vi "RemoteControl.vi"() -> ()   [LabVIEW 2019]
uses:
  <vilib>/ReMiSYS/ReMiSYS_WSCbot-XS/SubVI/XS_F710.ctl
  <vilib>/ReMiSYS/ReMiSYS_WSCbot-XS/SubVI/XS_stick.ctl
  <vilib>/ReMiSYS/ReMiSYS_WSCbot-XS/SubVI/XS_gamepadF710.lvclass
  WSCbot_V3_Toolkit.lvlibp/WSCBOTV3_Toolkit/IO/LowLevel/PulseCounter.ctl
  <vilib>/Platform/TimedLoop/XDataNode/timing_clust.ctl
  <vilib>/Platform/TimedLoop/XDataNode/nitl_modes.ctl
  <vilib>/Platform/TimedLoop/XDataNode/wakeup.ctl
  WSCbot_V3_Toolkit.lvlibp/WSCBOTV3_Toolkit/IO/LowLevel/IO_Chanel_DIO.ctl
  <vilib>/platform/TimedLoop/XDataNode/XDataNode.xnode
  <vilib>/Platform/TimedLoop/XDataNode/XDNodeRunTimeDep.lvlib
  WSCbot_V3_Toolkit.lvlibp
panel:
  out "PulseCount":i32
  out "Trun 180":bool
  out "positive":bool
  out "F710 button info.right":bool
  out "F710 button info.left":bool
  out "Angle_index":i32
  in  "Angle_array(deg)":dbl[](array[numeric])=[-65.0, 25.0, 115.0]
  out "F710 button info.LogiB":bool
  out "F710 button info.rightStick":bool
  out "EMS":bool
  in  "MaxSpeed":dbl=800.0
  out "H/L Speed":bool
  out "Current_High":dbl
  out "F710 button info.down":bool
  out "F710 button info.up":bool
  out "Flat":bool
  out "Home?":bool
  out "leftStick_Touch\nTimes":i8
  in  "High_array(mm)":dbl[](array[numeric])=[0.0, 78.0, 128.0, 250.0, 300.0]
  out "Hight":i32
  out "Front/Back":bool
  out "up":bool
  out "F710 button info.leftStick":bool
  out "F710 button info.B":bool
  out "F710 button info.X":bool
  out "F710 button info.A":bool
  out "F710 button info.Y":bool
  out "F710 button info.RB":bool
  out "F710 button info.LB":bool
  out "ini":bool
  out "reset":bool
  out "angle":dbl
  out "speed":dbl
  out "Error Out":errorcluster
  in  "Stop Button":bool
  in  "error in (no error)":errorcluster
  in  "INPUT S/N":string="U16N121E"
  in  "VISA resource name":refnum<visa-resource-name>="USB0::0x046D::0xC21F::145C9E1C::RAW"
  out "Stop Output":bool
  out "SpeedArray":dbl[](array[numeric])
  out "F710":T1
  # "螺絲物料櫃(1)\n螺絲物料櫃(2)\n螺帽物料櫃\n螺帽物料櫃瞄準"
  # "總高度300mm"
  # "朝左"
  # "朝前"
  # "朝右"
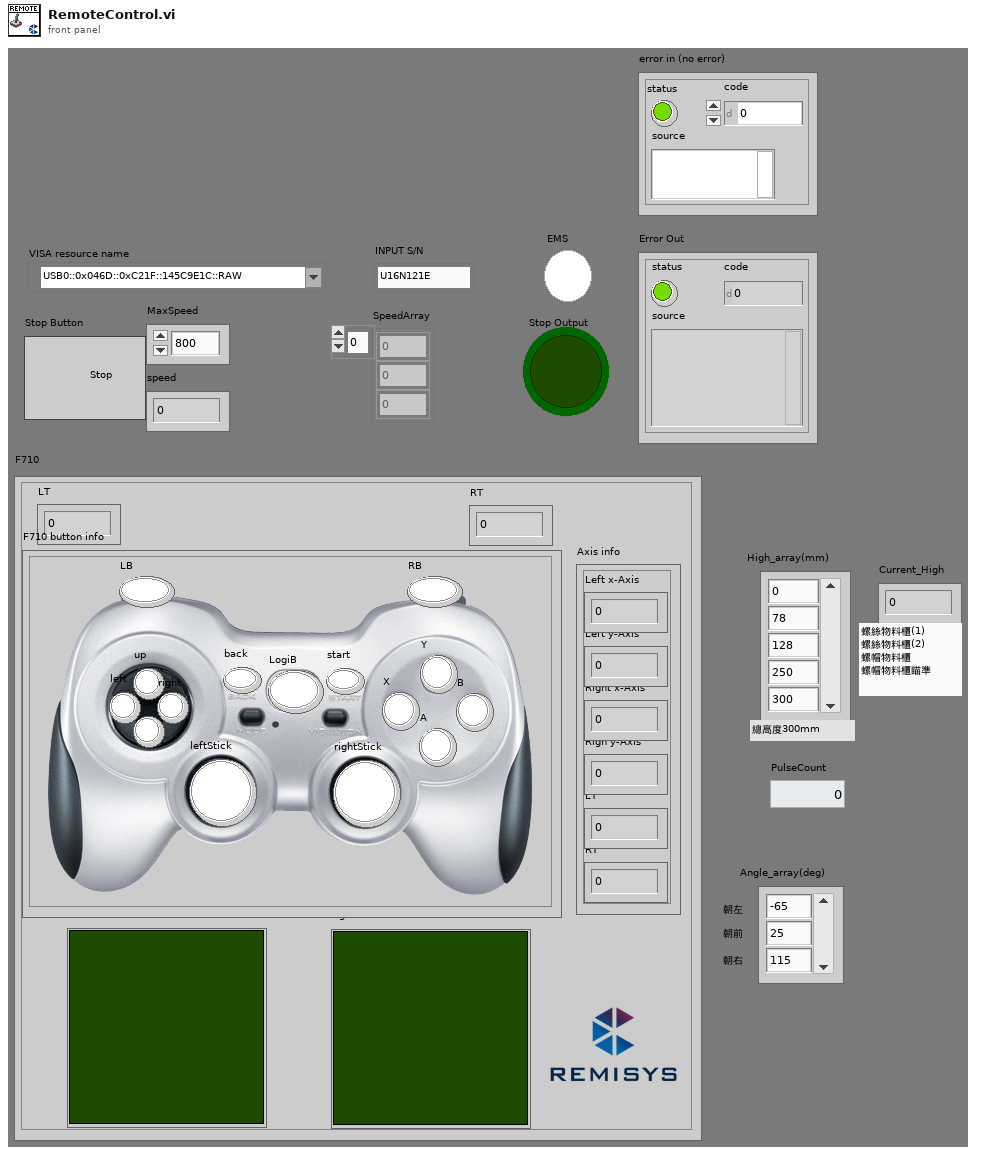
[diagram p1: front panel]
types:
  T1 = typedef "XS_F710.ctl" = cluster{"RT":u8, "LT":u8, "RightStick":T2, "LeftStick":T2, "Axis info":cluster{"Left x-Axis":i8, "Left y-Axis":i8, "Right x-Axis":i8, "Righ y-Axis":i8, "LT":u8, "RT":u8}, "F710 button info":cluster{"RB":bool, "LB":bool, "rightStick":bool, "leftStick":bool, "start":bool, "back":bool, "right":bool, "left":bool, "down":bool, "up":bool, "Y":bool, "X":bool, "B":bool, "A":bool, "LogiB":bool}}
  T2 = typedef "XS_stick.ctl" = cluster{"X":dbl, "Y":dbl}[]
  T3 = typedef "WSCbot_V3_Toolkit.lvlibp/PulseCounter.ctl" = enum16{"CH1", "CH2", "CH3", "CH4", "CH5"}
  T4 = typedef "WSCbot_V3_Toolkit.lvlibp/IO_Chanel_DIO.ctl" = enum16{"A/DIO9", "A/DIO10", "C/DIO0", "C/DIO1", "C/DIO2", "C/DIO3", "C/DIO4", "C/DIO5", "C/DIO6"}
  T5 = typedef "XDNodeRunTimeDep.lvlib/timing_clust.ctl" = cluster{"Expected End [f-1]":u64, "Actual End [f-1]":u64, "Finished Late? [f-1]":bool, "Expected End [i-1]":u64, "Actual End [i-1]":u64, "Finished Late? [i-1]":bool, "Expected Start [i]":u64, "Actual Start [i]":u64, "Expected Start [f]":u64, "Actual Start [f]":u64, "Source Name":string, "Structure Name":string, "Period":i64, "Deadline":i64, "Offset":i64, "Start":i64, "Priority":i32, "Timeout":i32, "Mode":T6, "Wakeup Reason":T7, "Error":errorcluster, "Source Type":string, "Secondary Source Type":string, "Global End Time":u64, "Global Start Time":u64, "Frame Duration":u64, "Iteration Duration":u64, "Assigned CPU":i32, "I/O Scan Engine Mode":u32}
  T6 = typedef "XDNodeRunTimeDep.lvlib/nitl_modes.ctl" = enum32{"No Change", "Process missed periods, maintain original phase", "Discard missed periods, maintain original phase", "Process missed periods, ignore original phase", "Discard missed periods, ignore original phase"}
  T7 = typedef "XDNodeRunTimeDep.lvlib/wakeup.ctl" = enum32{"Normal", "Aborted", "Asynchronous wakeup", "Timing source error", "Timed loop error", "Timeout"}
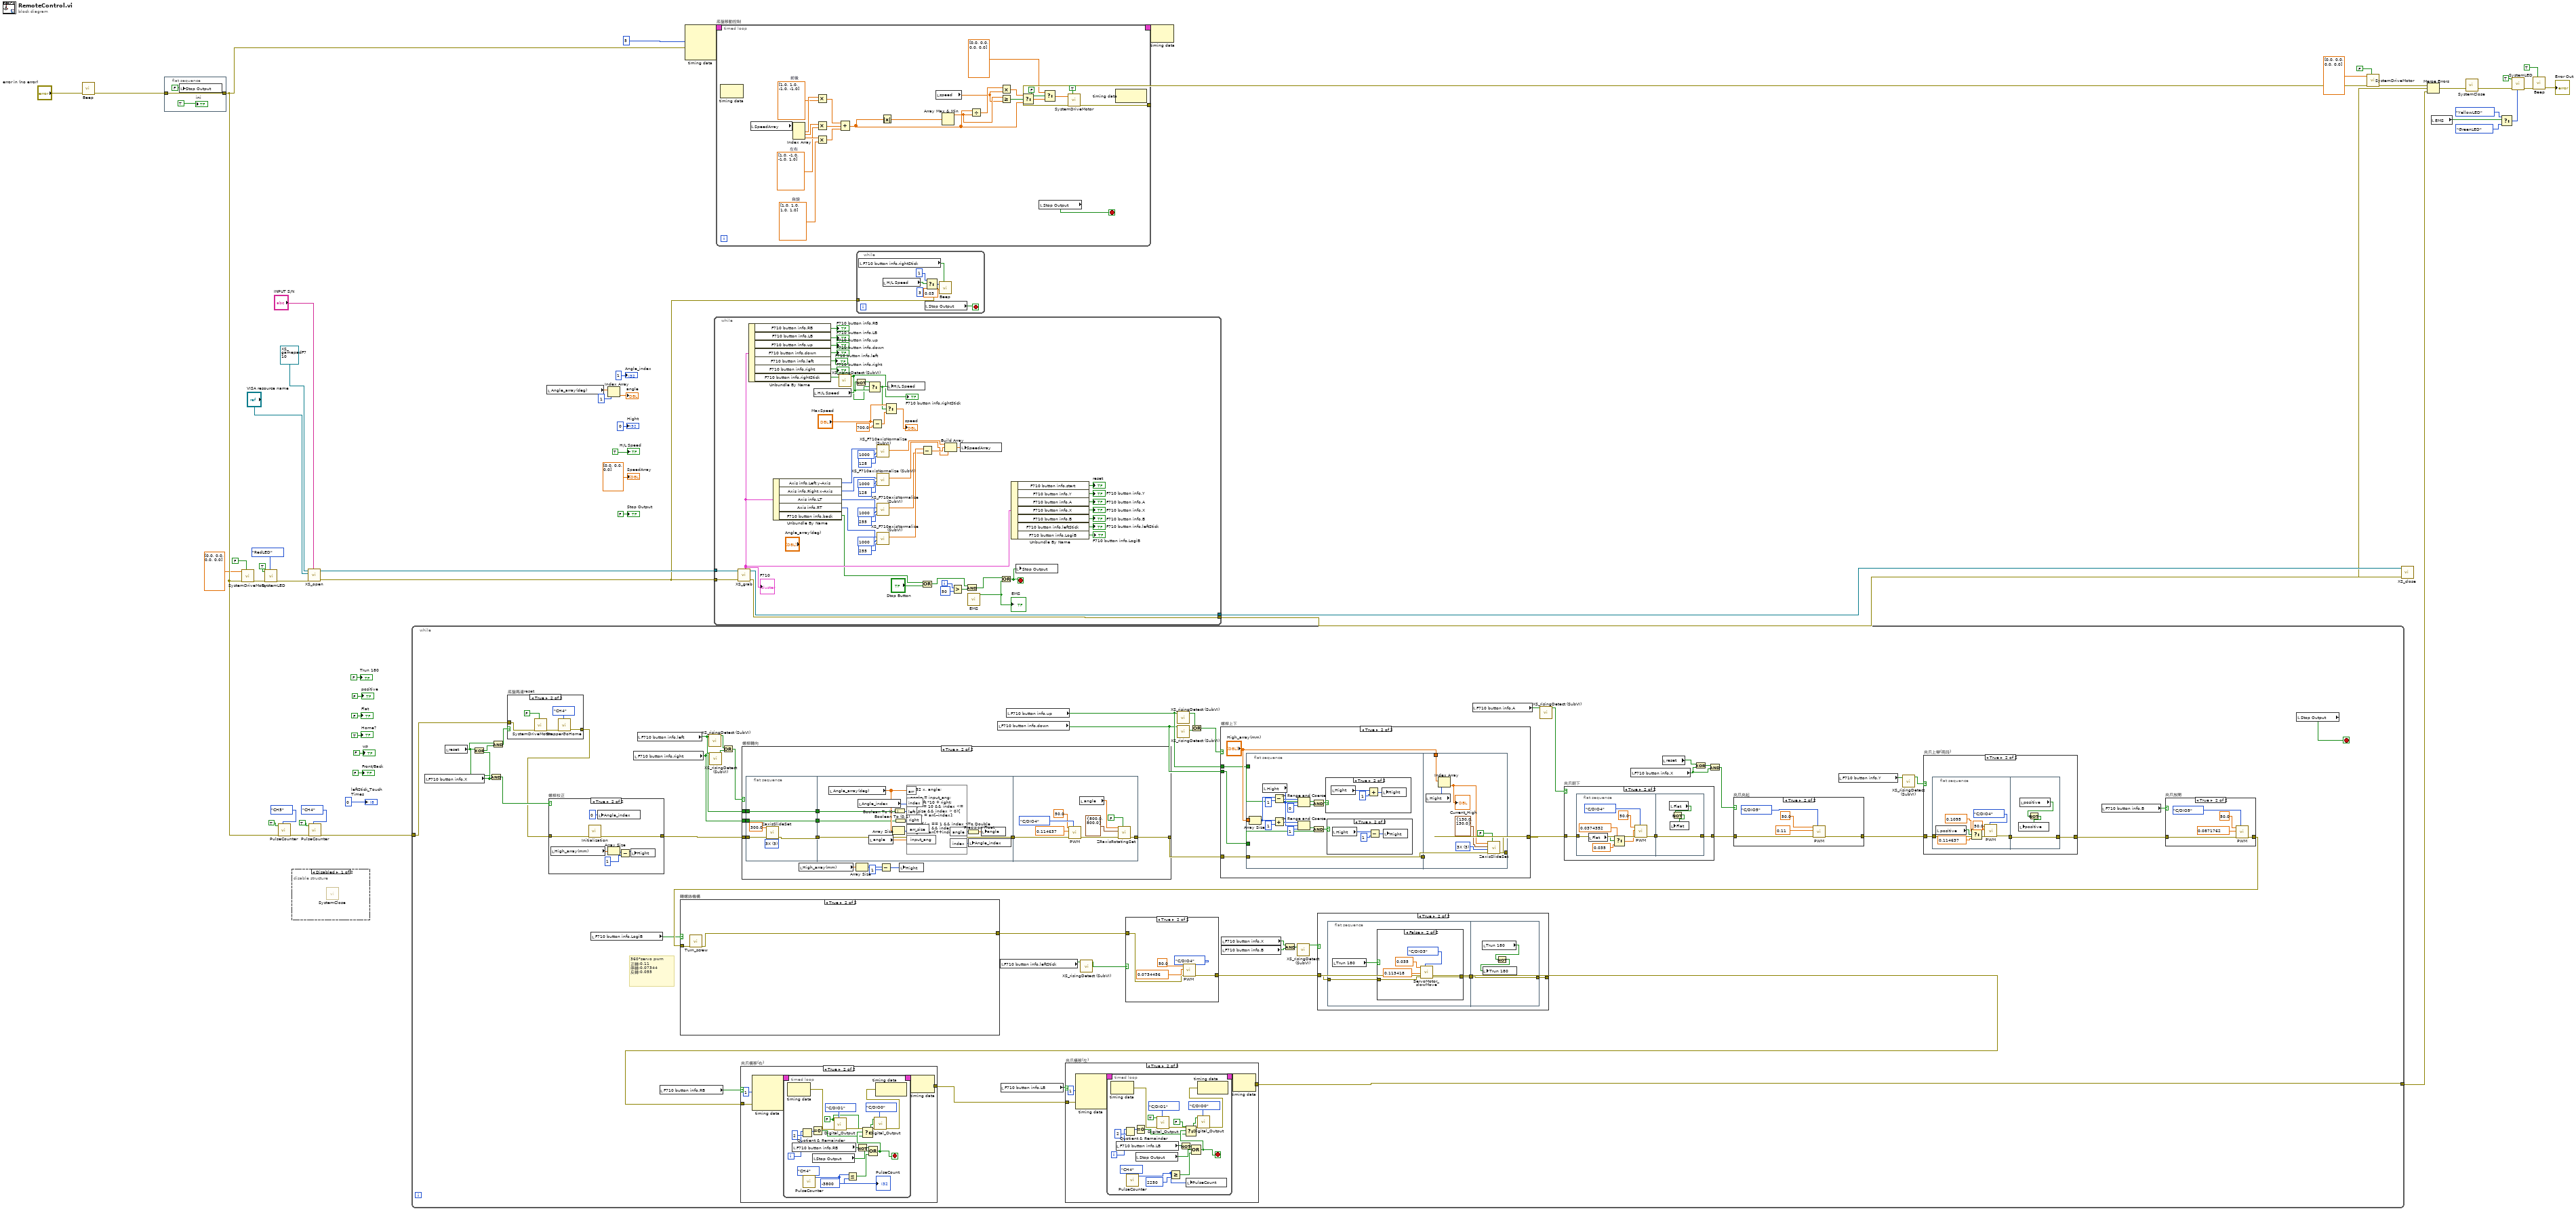
[diagram p0: block diagram]
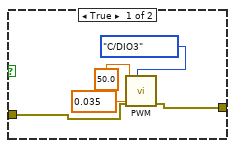
[diagram p4: hidden frame]
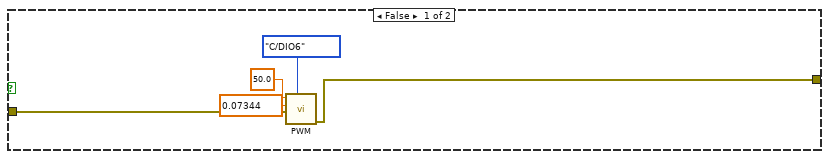
[diagram p8: hidden frame]
diagram:
  n1 = call "Beep.vi"("Error In"="error in (no error)") -> ("Error Out"=w17:errorcluster)  [unwired: 10 in]
  n2 = flat-sequence {
    tunnel: [w58] -> w35
    tunnel: w17 -> [w58]
    frame #0 {
      n3 = local write "Stop Output"(FALSE ("Stop Output")) -> ()
      "ini" <- TRUE
    }
  }
  n4 = call "SystemDriveMotor.vi"("Enable?"=FALSE, "error in"=w35, "4xMotor(deg/s)"=dbl[] [0.0, 0.0, 0.0, 0.0]) -> ("error out"=w46:errorcluster)  [unwired: 7 in, 1 out]
  n5 = call "SystemLED.vi"("SelectColor"=enum16{"RedLED", "GreenLED", "YellowLED"}."RedLED", "error in"=w46, "Set"=TRUE) -> ("error out"=w49:errorcluster)  [unwired: 8 in]
  n6 = call "PulseCounter.vi"("PulseCounterChanel"=PulseCounter."CH5", "error in"=w35, "Reset"=TRUE) -> ("error out"=w31:errorcluster)  [unwired: 7 in, 1 out]
  n7 = disable-structure shown="Disabled" {
    frame Disabled {
      n8 = call "SystemClose.vi"() -> ()  [unwired: 3 in, 1 out]
    }
    frame Enabled {
    }
  }
  n9 = call <vilib>:"XS_open.vi"("INPUT S/N"="INPUT S/N", "error in (no error)"=w49, "VISA resource name"="VISA resource name", "gamepadF710 in"=refnum<class "XS_gamepadF710.lvclass"> refnum) -> ("error out"=w14:errorcluster, "gamepadF710 out"=w50:refnum<class "XS_gamepadF710.lvclass">)  [unwired: 6 in]
  n10 = call "PulseCounter.vi"("PulseCounterChanel"=PulseCounter."CH4", "error in"=w31, "Reset"=TRUE) -> ("error out"=w30:errorcluster)  [unwired: 7 in, 1 out]
  n11 = while {
    tunnel: w30 -> [w94]
    tunnel: [w60] -> w36
    stop <- w106 stop-if-true
    # "360°servo pwm\n正轉:0.11\n停轉:0.07344\n反轉:0.055"
    n12 = local read "F710 button info.X"() -> (w103:bool)
    n13 = local read "reset"() -> (w86:bool)
    n14 = Exclusive Or(1:w103, 2:w86) -> (0:w87:bool)
    n15 = And(x=w86, y=w103) -> (x .and. y?=w104:bool)
    n16 = And(x=w86, y=w87) -> (x .and. y?=w88:bool)
    n17 = case "底盤馬達reset" shown="True" w88 {
      tunnel: w94 -> [w255 w257]
      tunnel: [w255 w256] -> w93
      frame False {
      }
      frame True {
        n18 = call "SystemDriveMotor.vi"("Enable?"=FALSE, "error in"=w257) -> ("error out"=w259:errorcluster)  [unwired: 8 in, 1 out]
        n19 = call "StepperGoHome.vi"("PulseCounterChanel"=PulseCounter."CH4", "Error In"=w259) -> ("Error Out"=w256:errorcluster)  [unwired: 7 in, 2 out]
      }
    }
    n20 = case "螺桿校正" shown="True" w104 {
      tunnel: w93 -> [w261 w268]
      tunnel: [w261 w266] -> w105
      frame False {
      }
      frame True {
        n21 = local read "High_array(mm)"() -> (w265:dbl[])
        n22 = call "Initialization.vi"("Error In"=w268) -> ("Error Out"=w266:errorcluster)  [unwired: 10 in]
        n23 = local write "Angle_index"(0 ("Hight")) -> ()
        n24 = Array Size(array=w265) -> (size(s)=w264:i32)
        n25 = Subtract(x=w264, y=1) -> (x-y=w262:i32)
        n26 = local write "Hight"(w262) -> ()
      }
    }
    n27 = local read "F710 button info.LogiB"() -> (w75:bool)
    n28 = local read "F710 button info.right"() -> (w70:bool)
    n29 = local read "F710 button info.left"() -> (w69:bool)
    n30 = local read "F710 button info.RB"() -> (w78:bool)
    n31 = call <vilib>:"XS_risingDetect (SubVI).vi"("y"=w69) -> ("Boolean"=w73:bool)  [unwired: 10 in]
    n32 = call <vilib>:"XS_risingDetect (SubVI).vi"("y"=w70) -> ("Boolean"=w72:bool)  [unwired: 10 in]
    n33 = Or(x=w73, y=w72) -> (x .or. y?=w71:bool)
    n34 = case "螺桿轉向" shown="True" w71 {
      tunnel: w105 -> [w306 w318]
      tunnel: [w306 w313] -> w99
      tunnel: w70 -> [_ w310]
      tunnel: w69 -> [_ w307]
      frame False {
      }
      frame True {
        n35 = flat-sequence {
          tunnel: w318 -> [w322]
          tunnel: [w319] -> w312
          tunnel: w310 -> [w321]
          tunnel: [w321] -> w309
          tunnel: [w320] -> w308
          tunnel: w307 -> [w320]
          tunnel: w312 -> [w336]
          tunnel: [w336] -> w311
          tunnel: w309 -> [w326]
          tunnel: w308 -> [w325]
          tunnel: w311 -> [w342]
          tunnel: [w338] -> w313
          frame #0 {
            w323 = u16 3 items=["0X", "1X", "2X", "3X"] ("findHomeVel (times)")
            n36 = call "ZaxisSlideSet.vi"("error in"=w322, "findHomeVel (times)"=w323, "TargetABSHight(mm)"=300.0) -> ("error out"=w319:errorcluster)  [unwired: 7 in, 1 out]
          }
          frame #1 {
            n37 = local read "Angle_array(deg)"() -> (w332:dbl[])
            n38 = local read "Angle_index"() -> (w333:i32)
            n39 = local read "angle"() -> (w327:dbl)
            n40 = Array Size(array=w332) -> (size(s)=w329:i32)
            n41 = Boolean To (0,1)(Boolean=w325) -> (0, 1=w335:i16)
            n42 = Boolean To (0,1)(Boolean=w326) -> (0, 1=w334:i16)
            n43 = formula code="int32 x, angle;\n\nangle = input_ang;\nx = left *10 + right;\nif (x == 10 && index <= arr_size && index > 0){\nangle = arr[--index];\n}\nelse if ( x == 1 && index < arr_size-1 && index >=0){\nangle = arr[++index];\n}"("left"=w335, "right"=w334, "index"=w333, "arr"=w332, "arr_size"=w329, "input_ang"=w327) -> ("angle"=w330:i32, "index"=w328:i32)
            n44 = To Double Precision Float(number=w330) -> (double precision float=w331:dbl)
            n45 = local write "Angle_index"(w328) -> ()
            n46 = local write "angle"(w331) -> ()
          }
          frame #2 {
            n47 = call "PWM.vi"("IO_Chanel"=IO_Chanel_DIO."C/DIO4", "error in"=w342, "DutyCycle"=0.114637, "Frequency(Hz)"=50.0) -> ("error out"=w341:errorcluster)  [unwired: 7 in]
            n48 = local read "angle"() -> (w337:dbl)
            n49 = call "ZRaxisRotatingSet.vi"("Reset"=FALSE, "error in"=w341, "Velocity(deg/s)&ACC(deg/ss)"=cluster{"Velocity(cm/s)":dbl, "ACC(cm/ss)":dbl} {"Velocity(cm/s)"=800.0, "ACC(cm/ss)"=800.0}, "TargetHight(deg)"=w337) -> ("error out"=w338:errorcluster)  [unwired: 6 in, 1 out]
          }
        }
        n50 = local read "High_array(mm)"() -> (w317:dbl[])
        n51 = Array Size(array=w317) -> (size(s)=w316:i32)
        n52 = Subtract(x=w316, y=1) -> (x-y=w314:i32)
        n53 = local write "Hight"(w314) -> ()
      }
    }
    n54 = local read "F710 button info.down"() -> (w79:bool)
    n55 = local read "F710 button info.leftStick"() -> (w68:bool)
    n56 = local read "F710 button info.LB"() -> (w77:bool)
    n57 = local read "F710 button info.up"() -> (w80:bool)
    n58 = call <vilib>:"XS_risingDetect (SubVI).vi"("y"=w68) -> ("Boolean"=w67:bool)  [unwired: 10 in]
    n59 = call <vilib>:"XS_risingDetect (SubVI).vi"("y"=w80) -> ("Boolean"=w76:bool)  [unwired: 10 in]
    n60 = call <vilib>:"XS_risingDetect (SubVI).vi"("y"=w79) -> ("Boolean"=w81:bool)  [unwired: 10 in]
    n61 = Or(x=w76, y=w81) -> (x .or. y?=w74:bool)
    n62 = case "螺桿上下" shown="True" w74 {
      tunnel: [w269 w273] -> w98
      tunnel: w99 -> [w269 w275]
      tunnel: w80 -> [_ w271]
      tunnel: w79 -> [_ w270]
      frame False {
      }
      frame True {
        n63 = flat-sequence {
          tunnel: "High_array(mm)" -> [w279]
          tunnel: w275 -> [w278]
          tunnel: [w278] -> w274
          tunnel: w271 -> [w277]
          tunnel: w270 -> [w276]
          tunnel: w274 -> [w300]
          tunnel: [w299] -> w273
          tunnel: "High_array(mm)" -> [w298]
          frame #0 {
            n64 = Array Size(array=w279) -> (size(s)=w289:i32)
            n65 = local read "Hight"() -> (w286:i32)
            n66 = Subtract(x=w289, y=1) -> (x-y=w291:i32)
            n67 = Add(x=w289, y=1) -> (x+y=w287:i32)
            n68 = In Range and Coerce(upper limit=w291, x=w286, lower limit=0) -> (In Range?=w285:bool)  [unwired: 1 out]
            n69 = In Range and Coerce(upper limit=w287, x=w286, lower limit=1) -> (In Range?=w283:bool)  [unwired: 1 out]
            n70 = And(x=w277, y=w285) -> (x .and. y?=w282:bool)
            n71 = And(x=w283, y=w276) -> (x .and. y?=w281:bool)
            n72 = case shown="True" w282 {
              frame False {
              }
              frame True {
                n73 = local read "Hight"() -> (w294:i32)
                n74 = Add(x=w294, y=1) -> (x+y=w293:i32)
                n75 = local write "Hight"(w293) -> ()
              }
            }
            n76 = case shown="True" w281 {
              frame False {
              }
              frame True {
                n77 = local read "Hight"() -> (w297:i32)
                n78 = Subtract(x=w297, y=1) -> (x-y=w296:i32)
                n79 = local write "Hight"(w296) -> ()
              }
            }
          }
          frame #1 {
            w302 = u16 3 items=["0X", "1X", "2X", "3X"] ("findHomeVel (times)")
            n80 = local read "Hight"() -> (w304:i32)
            n81 = Index Array(array=w298, index=w304) -> (element=w305:dbl)
            "Current_High" <- w305
            n82 = call "ZaxisSlideSet.vi"("Reset"=FALSE, "error in"=w300, "findHomeVel (times)"=w302, "Velocity(mm/s)&ACC(mm/ss)"=cluster{"Velocity(cm/s)":dbl, "ACC(cm/ss)":dbl} {"Velocity(cm/s)"=130.0, "ACC(cm/ss)"=130.0}, "TargetABSHight(mm)"=w305) -> ("error out"=w299:errorcluster)  [unwired: 5 in, 1 out]
          }
        }
      }
    }
    n83 = local read "F710 button info.X"() -> (w64:bool)
    n84 = local read "F710 button info.B"() -> (w63:bool)
    n85 = And(x=w64, y=w63) -> (x .and. y?=w62:bool)
    n86 = call <vilib>:"XS_risingDetect (SubVI).vi"("y"=w62) -> ("Boolean"=w61:bool)  [unwired: 10 in]
    n87 = local read "F710 button info.A"() -> (w83:bool)
    n88 = call <vilib>:"XS_risingDetect (SubVI).vi"("y"=w83) -> ("Boolean"=w82:bool)  [unwired: 10 in]
    n89 = case "夾爪朝下" shown="True" w82 {
      tunnel: [w225 w228] -> w101
      tunnel: w98 -> [w225 w227]
      frame False {
      }
      frame True {
        n90 = flat-sequence {
          tunnel: w227 -> [w233]
          tunnel: [w234] -> w226
          tunnel: [w239] -> w228
          tunnel: w226 -> [w239]
          frame #0 {
            n91 = local read "Flat"() -> (w230:bool)
            n92 = Select(t=0.0374352, s=w230, f=0.035 ("DutyCycle")) -> (s? t:f=w231:dbl)
            n93 = call "PWM.vi"("IO_Chanel"=IO_Chanel_DIO."C/DIO4", "error in"=w233, "DutyCycle"=w231, "Frequency(Hz)"=50.0) -> ("error out"=w234:errorcluster)  [unwired: 7 in]
          }
          frame #1 {
            n94 = local read "Flat"() -> (w237:bool)
            n95 = Not(x=w237) -> (.not. x?=w238:bool)
            n96 = local write "Flat"(w238) -> ()
          }
        }
      }
    }
    n97 = local read "F710 button info.X"() -> (w90:bool)
    n98 = local read "reset"() -> (w89:bool)
    n99 = Exclusive Or(1:w90, 2:w89) -> (0:w92:bool)
    n100 = And(x=w92, y=w90) -> (x .and. y?=w91:bool)
    n101 = case "夾爪夾起" shown="True" w91 {
      tunnel: w101 -> [w213 w215]
      tunnel: [w213 w214] -> w97
      frame False {
      }
      frame True {
        n102 = call "PWM.vi"("IO_Chanel"=IO_Chanel_DIO."C/DIO5", "error in"=w215, "DutyCycle"=0.11, "Frequency(Hz)"=50.0) -> ("error out"=w214:errorcluster)  [unwired: 7 in]
      }
    }
    n103 = local read "F710 button info.Y"() -> (w85:bool)
    n104 = call <vilib>:"XS_risingDetect (SubVI).vi"("y"=w85) -> ("Boolean"=w84:bool)  [unwired: 10 in]
    n105 = case "夾爪上舉(兩段)" shown="True" w84 {
      tunnel: [w240 w242] -> w102
      tunnel: w97 -> [w240 w243]
      frame False {
      }
      frame True {
        n106 = flat-sequence {
          tunnel: w243 -> [w249]
          tunnel: [w248] -> w241
          tunnel: [w254] -> w242
          tunnel: w241 -> [w254]
          frame #0 {
            n107 = local read "positive"() -> (w245:bool)
            n108 = Select(t=0.1095 ("DutyCycle"), s=w245, f=0.114637 ("DutyCycle")) -> (s? t:f=w247:dbl)
            n109 = call "PWM.vi"("IO_Chanel"=IO_Chanel_DIO."C/DIO4", "error in"=w249, "DutyCycle"=w247, "Frequency(Hz)"=50.0) -> ("error out"=w248:errorcluster)  [unwired: 7 in]
          }
          frame #1 {
            n110 = local read "positive"() -> (w253:bool)
            n111 = Not(x=w253) -> (.not. x?=w252:bool)
            n112 = local write "positive"(w252) -> ()
          }
        }
      }
    }
    n113 = local read "F710 button info.B"() -> (w100:bool)
    n114 = case "夾爪放開" shown="True" w100 {
      tunnel: w102 -> [w219 w221]
      tunnel: [w219 w220] -> w96
      frame False {
      }
      frame True {
        n115 = call "PWM.vi"("IO_Chanel"=IO_Chanel_DIO."C/DIO5", "error in"=w221, "DutyCycle"=0.0871762, "Frequency(Hz)"=50.0) -> ("error out"=w220:errorcluster)  [unwired: 7 in]
      }
    }
    n116 = case "轉螺絲機構" shown="True" w75 {
      tunnel: w96 -> [w207 w212]
      tunnel: [w206 w211] -> w66
      frame False {
        n117 = call "PWM.vi"("IO_Chanel"=IO_Chanel_DIO."C/DIO6", "error in"=w207, "DutyCycle"=0.07344, "Frequency(Hz)"=50.0) -> ("error out"=w206:errorcluster)  [unwired: 7 in]
      }
      frame True {
        n118 = call "Turn_screw.vi"("Error In"=w212) -> ("Error Out"=w211:errorcluster)  [unwired: 10 in]
      }
    }
    n119 = case shown="True" w67 {
      tunnel: w66 -> [w127 w130]
      tunnel: [w127 w129] -> w65
      frame False {
      }
      frame True {
        n120 = call "PWM.vi"("IO_Chanel"=IO_Chanel_DIO."C/DIO4", "error in"=w130, "DutyCycle"=0.0734456, "Frequency(Hz)"=50.0) -> ("error out"=w129:errorcluster)  [unwired: 7 in]
      }
    }
    n121 = case "夾爪橫移(右)" shown="True" w78 {
      tunnel: w65 -> [w170 w172]
      tunnel: [w170 w171] -> w95
      frame False {
      }
      frame True {
        n122 = node-c288(i64 1 ("Period"), w172) -> (w175:T5)  [unwired: 2 in]
        n123 = timed-loop {
          timing: w175 -> [_]
          timing-out: [_] -> w174
          i -> [w189]
          stop <- w179 stop-if-true
          w177 = FALSE ("False/True")
          n124 = node-c288() -> (w185:errorcluster)  [unwired: 1 in]
          n125 = local read "F710 button info.RB"() -> (w188:bool)
          n126 = Quotient & Remainder(x=w189, y=2) -> (x-y*floor(x/y)=w190:i32)  [unwired: 1 out]
          n127 = call "PulseCounter.vi"("PulseCounterChanel"=PulseCounter."CH4") -> ("PulseCount"=w182:i32)  [unwired: 9 in, 1 out]
          "PulseCount" <- w182
          n128 = Equal To 0?(x=w190) -> (x = 0?=w178:bool)
          n129 = local read "Stop Output"() -> (w186:bool)
          n130 = call "Digital_Output.vi"("IO_Chanel"=IO_Chanel_DIO."C/DIO1", "error in"=w185, "False/True"=w177) -> ("error out"=w193:errorcluster)  [unwired: 8 in]
          n131 = Less Or Equal?(x=w182, y=-3800) -> (x <= y?=w180:bool)
          n132 = Not(x=w188) -> (.not. x?=w187:bool)
          n133 = Compound Arithmetic op=OR(w187, w186, w180) -> (w179:bool)
          n134 = Select(t=w177, s=w179, f=w178) -> (s? t:f=w176:bool)
          n135 = call "Digital_Output.vi"("IO_Chanel"=IO_Chanel_DIO."C/DIO0", "error in"=w193, "False/True"=w176) -> ("error out"=w184:errorcluster)  [unwired: 8 in]
          n136 = node-c288(w184) -> ()  [unwired: 1 out]
        }
        n137 = node-c288(w174) -> (w171:errorcluster)
      }
    }
    n138 = case "夾爪橫移(左)" shown="True" w77 {
      tunnel: w95 -> [w133 w136]
      tunnel: [w133 w135] -> w60
      frame False {
      }
      frame True {
        n139 = node-c288(i64 1 ("Period"), w136) -> (w138:T5)  [unwired: 2 in]
        n140 = timed-loop {
          timing: w138 -> [_]
          timing-out: [_] -> w137
          i -> [w153]
          stop <- w144 stop-if-true
          n141 = node-c288() -> (w149:errorcluster)  [unwired: 1 in]
          n142 = local read "F710 button info.LB"() -> (w152:bool)
          n143 = Quotient & Remainder(x=w153, y=2) -> (x-y*floor(x/y)=w154:i32)  [unwired: 1 out]
          n144 = call "PulseCounter.vi"("PulseCounterChanel"=PulseCounter."CH4") -> ("PulseCount"=w139:i32)  [unwired: 9 in, 1 out]
          n145 = Equal To 0?(x=w154) -> (x = 0?=w143:bool)
          n146 = local read "Stop Output"() -> (w150:bool)
          n147 = call "Digital_Output.vi"("IO_Chanel"=IO_Chanel_DIO."C/DIO1", "error in"=w149, "False/True"=TRUE) -> ("error out"=w157:errorcluster)  [unwired: 8 in]
          n148 = Greater Or Equal?(x=w139, y=2250) -> (x >= y?=w145:bool)
          n149 = Not(x=w152) -> (.not. x?=w151:bool)
          n150 = local write "PulseCount"(w139) -> ()
          n151 = Compound Arithmetic op=OR(w151, w150, w145) -> (w144:bool)
          n152 = Select(t=FALSE, s=w144, f=w143) -> (s? t:f=w141:bool)
          n153 = call "Digital_Output.vi"("IO_Chanel"=IO_Chanel_DIO."C/DIO0", "error in"=w157, "False/True"=w141) -> ("error out"=w148:errorcluster)  [unwired: 8 in]
          n154 = node-c288(w148) -> ()  [unwired: 1 out]
        }
        n155 = node-c288(w137) -> (w135:errorcluster)
      }
    }
    n156 = case shown="True" w61 {
      tunnel: w65 -> [w107 w110]
      tunnel: [w107 w108] -> _
      frame False {
      }
      frame True {
        n157 = flat-sequence {
          tunnel: w110 -> [w112]
          tunnel: [w111] -> w109
          tunnel: w109 -> [w124]
          tunnel: [w124] -> w108
          frame #0 {
            n158 = local read "Trun 180"() -> (w113:bool)
            n159 = case shown="False" w113 {
              tunnel: w112 -> [w114 w120]
              tunnel: [w115 w119] -> w111
              frame True {
                n160 = call "PWM.vi"("IO_Chanel"=IO_Chanel_DIO."C/DIO3", "error in"=w114, "DutyCycle"=0.035, "Frequency(Hz)"=50.0) -> ("error out"=w115:errorcluster)  [unwired: 7 in]
              }
              frame False {
                n161 = call "ServoMotor_slowMove.vi"("IO_Chanel"=IO_Chanel_DIO."C/DIO3", "Error In"=w120, "pwm_target"=0.113418, "pwm_start"=0.035) -> ("Error Out"=w119:errorcluster)  [unwired: 7 in]
              }
            }
          }
          frame #1 {
            n162 = local read "Trun 180"() -> (w126:bool)
            n163 = Not(x=w126) -> (.not. x?=w125:bool)
            n164 = local write "Trun 180"(w125) -> ()
          }
        }
      }
    }
    n165 = local read "Stop Output"() -> (w106:bool)
  }
  n166 = local read "Angle_array(deg)"() -> (w5:dbl[])
  n167 = Index Array(array=w5, index=1) -> (element=→"angle":dbl)
  n168 = node-c288(i64 5 ("Period"), w35) -> (w56:T5)  [unwired: 2 in]
  n169 = while {
    tunnel: w50 -> [w399]
    tunnel: [w398] -> w52
    tunnel: [w388] -> w20
    tunnel: w14 -> [w387]
    i -> [w386]
    stop <- w349 stop-if-true
    n170 = call <vilib>:"XS_grab.vi"("error in (no error)"=w387, "gamepadF710 in"=w399) -> ("error out"=w388:errorcluster, "gamepadF710 out"=w398:refnum<class "XS_gamepadF710.lvclass">, "F710"=w372:T1)  [unwired: 6 in]
    "F710" <- w372
    n171 = Unbundle By Name(w372) -> ("F710 button info.RB"=→"F710 button info.RB":bool, "F710 button info.LB"=→"F710 button info.LB":bool, "F710 button info.up"=→"F710 button info.up":bool, "F710 button info.down"=→"F710 button info.down":bool, "F710 button info.left"=→"F710 button info.left":bool, "F710 button info.right"=→"F710 button info.right":bool, "F710 button info.rightStick"=w365:bool)
    n172 = Unbundle By Name(w372) -> ("Axis info.Left y-Axis"=w381:i8, "Axis info.Right x-Axis"=w380:i8, "Axis info.LT"=w379:u8, "Axis info.RT"=w378:u8, "F710 button info.back"=w352:bool)
    n173 = local read "H/L Speed"() -> (w363:bool)
    n174 = call <vilib>:"XS_risingDetect (SubVI).vi"("y"=w365) -> ("Boolean"=w353:bool)  [unwired: 10 in]
    "F710 button info.rightStick" <- w353
    n175 = Not(x=w363) -> (.not. x?=w348:bool)
    n176 = Select(t=w348, s=w353, f=w363) -> (s? t:f=w354:bool)
    n177 = Subtract(x="MaxSpeed", y=700.0) -> (x-y=w361:dbl)
    n178 = call <vilib>:"XS_F710axisNormalize (SubVI).vi"("rawRange"=128, "normalizeTo"=1000, "axisInput"=w381) -> ("NormalizedValue"=w389:dbl)  [unwired: 8 in]
    n179 = call <vilib>:"XS_F710axisNormalize (SubVI).vi"("rawRange"=128, "normalizeTo"=1000, "axisInput"=w380) -> ("NormalizedValue"=w376:dbl)  [unwired: 8 in]
    n180 = call <vilib>:"XS_F710axisNormalize (SubVI).vi"("rawRange"=255, "normalizeTo"=1000, "axisInput"=w379) -> ("NormalizedValue"=w374:dbl)  [unwired: 8 in]
    n181 = call <vilib>:"XS_F710axisNormalize (SubVI).vi"("rawRange"=255, "normalizeTo"=1000, "axisInput"=w378) -> ("NormalizedValue"=w375:dbl)  [unwired: 8 in]
    n182 = Select(t="MaxSpeed", s=w354, f=w361) -> (s? t:f=→"speed":dbl)
    n183 = local write "H/L Speed"(w354) -> ()
    n184 = Subtract(x=w375, y=w374) -> (x-y=w377:dbl)
    n185 = Compound Arithmetic op=OR(w352, "Stop Button") -> (w383:bool)
    n186 = Build Array(w389, w377, w376) -> (w351:dbl[])
    n187 = Greater?(x=w386, y=50) -> (0:w384:bool)
    n188 = local write "SpeedArray"(w351) -> ()
    n189 = And(x=w383, y=w384) -> (x .and. y?=w369:bool)
    n190 = call "EMS.vi"() -> ("EMS"=w355:bool)  [unwired: 10 in, 1 out]
    "EMS" <- w355
    n191 = Or(x=w369, y=w355) -> (x .or. y?=w349:bool)
    n192 = Unbundle By Name(w372) -> ("F710 button info.start"=→"reset":bool, "F710 button info.Y"=→"F710 button info.Y":bool, "F710 button info.A"=→"F710 button info.A":bool, "F710 button info.X"=→"F710 button info.X":bool, "F710 button info.B"=→"F710 button info.B":bool, "F710 button info.leftStick"=→"F710 button info.leftStick":bool, "F710 button info.LogiB"=→"F710 button info.LogiB":bool)
    n193 = local write "Stop Output"(w349) -> ()
  }
  n194 = timed-loop "底盤移動控制" {
    timing: w56 -> [_]
    timing-out: [_] -> w55
    tunnel: [w407] -> w44
    stop <- w412 stop-if-true
    w423 = dbl[] [1.0, 1.0, 1.0, 1.0]  # 自旋
    w401 = dbl[] [1.0, -1.0, -1.0, 1.0]  # 左右
    w402 = dbl[] [1.0, 1.0, -1.0, -1.0]  # 前後
    n195 = node-c288() -> ()  [unwired: 1 in, 1 out]
    n196 = local read "SpeedArray"() -> (w416:dbl[])
    n197 = Index Array(array=w416) -> (element #1=w404:dbl, element #2=w400:dbl, element #3=w403:dbl)  [unwired: 3 in]
    n198 = Multiply(x=w404, y=w402) -> (x*y=w422:dbl[])
    n199 = Multiply(x=w400, y=w401) -> (x*y=w421:dbl[])
    n200 = Multiply(x=w403, y=w423) -> (x*y=w420:dbl[])
    n201 = Compound Arithmetic op=ADD(w422, w421, w420) -> (w417:dbl[])
    n202 = Absolute Value(x=w417) -> (abs(x)=w419:dbl[])
    n203 = local read "speed"() -> (w405:dbl)
    n204 = Array Max & Min(array=w419) -> (max value=w413:dbl)  [unwired: 3 out]
    n205 = Divide(x=w417, y=w413) -> (x/y=w415:dbl[])
    n206 = Multiply(x=w415, y=w405) -> (x*y=w414:dbl[])
    n207 = Greater Or Equal?(x=w413, y=w405) -> (x >= y?=w418:bool)
    n208 = Select(t=w414, s=w418, f=w417) -> (s? t:f=w411:dbl[])
    n209 = local read "Stop Output"() -> (w412:bool)
    n210 = Select(t=dbl[] [0.0, 0.0, 0.0, 0.0], s=FALSE, f=w411) -> (s? t:f=w409:dbl[])
    n211 = call "SystemDriveMotor.vi"("Enable?"=TRUE, "4xMotor(deg/s)"=w409) -> ("error out"=w407:errorcluster)  [unwired: 8 in, 1 out]
    n212 = node-c288() -> ()  [unwired: 1 in, 1 out]
  }
  n213 = while {
    tunnel: w14 -> [w427]
    stop <- w429 stop-if-true
    n214 = local read "F710 button info.rightStick"() -> (w426:bool)
    n215 = local read "H/L Speed"() -> (w428:bool)
    n216 = local read "Stop Output"() -> (w429:bool)
    n217 = Select(t=1, s=w428, f=3 ("Beep * n?")) -> (s? t:f=w433:i32)
    n218 = call "Beep.vi"("Enable"=w426, "Error In"=w427, "Beep duration\n(sec)"=0.03 ("Beep duration\n(sec)"), "Beep * n?"=w433) -> ()  [unwired: 7 in, 1 out]
  }
  n219 = node-c288(w55) -> ()  [unwired: 1 out]
  n220 = call "SystemDriveMotor.vi"("Enable?"=FALSE, "error in"=w44, "4xMotor(deg/s)"=dbl[] [0.0, 0.0, 0.0, 0.0]) -> ("error out"=w43:errorcluster)  [unwired: 7 in, 1 out]
  n221 = call <vilib>:"XS_close.vi"("error in (no error)"=w20, "gamepadF710 in"=w52) -> ("error out"=w25:errorcluster)  [unwired: 8 in, 1 out]
  n222 = Merge Errors(w43, w25, w36) -> (w16:errorcluster)
  n223 = local read "EMS"() -> (w18:bool)
  n224 = call "SystemClose.vi"("error in"=w16) -> ("error out"=w19:errorcluster)  [unwired: 2 in]
  n225 = Select(t=enum16{"RedLED", "GreenLED", "YellowLED"}."YellowLED" ("SelectColor"), s=w18, f=enum16{"RedLED", "GreenLED", "YellowLED"}."GreenLED" ("SelectColor")) -> (s? t:f=w23:enum16{"RedLED", "GreenLED", "YellowLED"})
  n226 = call "SystemLED.vi"("SelectColor"=w23, "error in"=w19, "Set"=TRUE) -> ("error out"=w11:errorcluster)  [unwired: 8 in]
  n227 = call "Beep.vi"("Enable"=TRUE, "Error In"=w11) -> ("Error Out"=→"Error Out":errorcluster)  [unwired: 9 in]
  "Front/Back" <- FALSE ("Boolean")
  "Hight" <- 0 ("Hight")
  "up" <- FALSE ("up")
  "leftStick_Touch\nTimes" <- i8 0 ("leftStick_Touch\nTimes")
  "Home?" <- TRUE ("First Time")
  "Flat" <- FALSE ("up")
  "H/L Speed" <- TRUE ("H/L Speed")
  "SpeedArray" <- dbl[] [0.0, 0.0, 0.0] ("SpeedArray")
  "Stop Output" <- FALSE ("Stop Output")
  "Angle_index" <- 1 ("Angle_index")
  "positive" <- FALSE ("positive")
  "Trun 180" <- FALSE ("Boolean")
